vi "GOOP_Utility_IsClassVI.vi"(7 "KeepClassOpen(False)":bool, 8 "error in (no error)":errorcluster, 10 "ProjectItem":refnum<vi>, 11 "Object":u64) -> (0 "error out":errorcluster, 1 "ClassItem(If Found)":refnum<vi>, 2 "ClassProvider":string, 3 "Is Class VI?":bool, 4 "RootClassQualified Class Name":string, 5 "Is Interface?":bool)   [LabVIEW 2020]
uses:
  <resource>/Framework/Providers/Open_GDS/ClassProviders/Common/LvClass_class/GDSLvClass_ClassTypeSettingNames.ctl
  <resource>/Framework/Providers/Open_GDS/ClassProviders/Provider_LvNativeClass/LvNativeProviderName.ctl
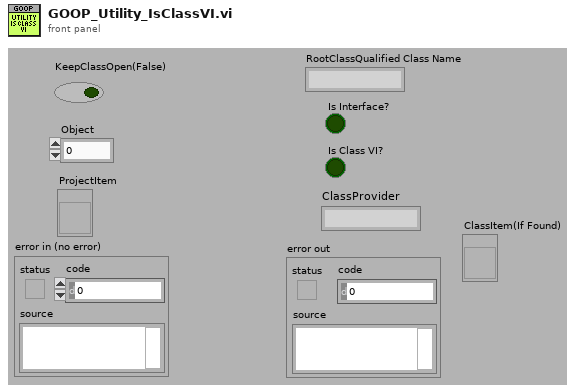
[diagram p1: front panel]
types:
  T1 = typedef "LvNativeProviderName.ctl" = enum16{"Endevo LabVIEW Native"}
  T2 = typedef "GDSLvClass_ClassTypeSettingNames.ctl" = enum16{"EndevoGOOP_ClassProvider", "EndevoGOOP_TemplateUsed", "EndevoGOOP_TemplateVersion", "EndevoGOOP_PlugIns", "EndevoGOOP_ConnectorPanePattern"}
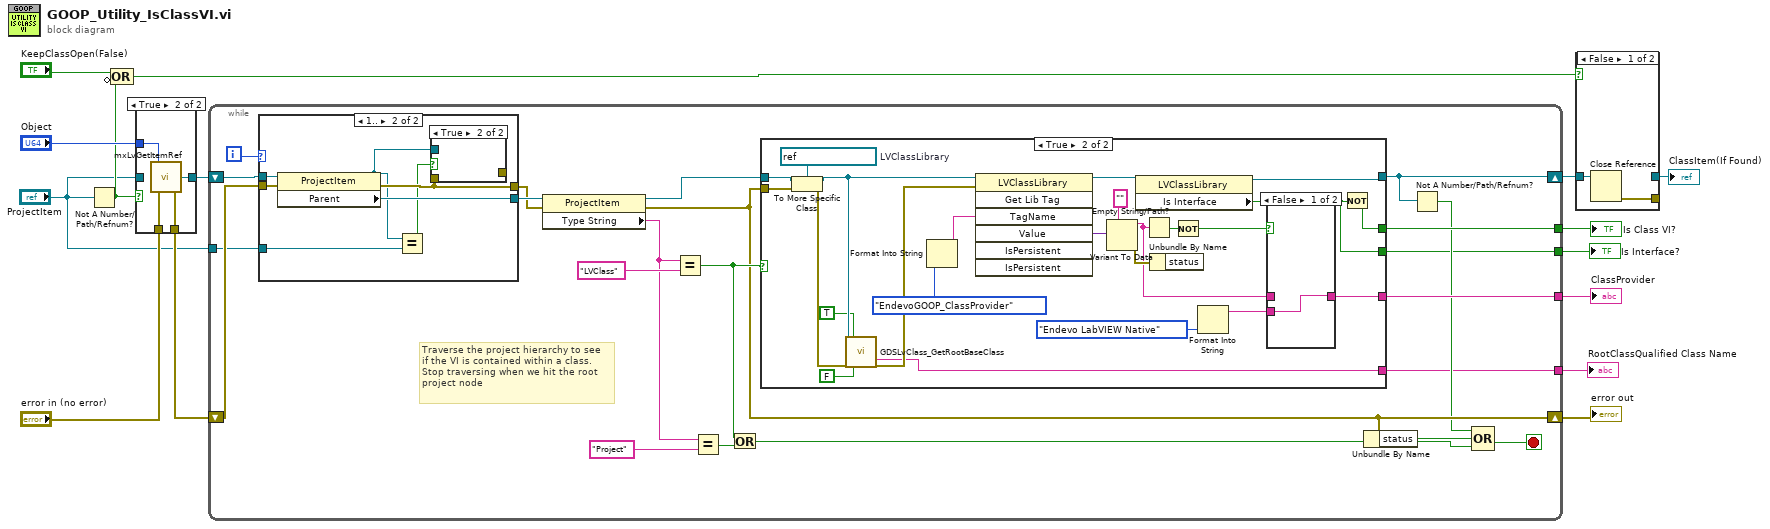
[diagram p0: block diagram]
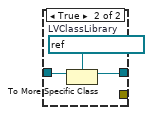
[diagram p3: hidden frame]
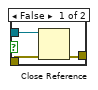
[diagram p5: hidden frame]
diagram:
  n1 = Not A Number/Path/Refnum?(number/path/refnum="ProjectItem") -> (NaN/Path/Refnum?=w4:bool)
  n2 = Compound Arithmetic op=OR("KeepClassOpen(False)", invert w4) -> (w5:bool)
  n3 = case shown="True" w4 {
    tunnel: "Object" -> [_ w21]
    tunnel: [w16 w20] -> w14
    tunnel: "error in (no error)" -> [w17 w19]
    tunnel: [w17 w18] -> w10
    tunnel: "ProjectItem" -> [w16 _]
    frame False {
    }
    frame True {
      n4 = call <resource>:"mxLvGetItemRef.vi"("Item"=w21, "error in"=w19) -> ("Item Refnum"=w20:refnum<vi>, "error out"=w18:errorcluster)  [unwired: 1 out]
    }
  }
  n5 = while {
    shift-right: [w29] -> w8
    shift-left: w14 -> [w41]
    tunnel: [w35] -> w13
    tunnel: [w34] -> w11
    shift-right: [w30] -> w9
    shift-left: w10 -> [w33]
    tunnel: "ProjectItem" -> [w24]
    tunnel: [w23] -> w2
    tunnel: [w22] -> w1
    i -> [w31]
    stop <- w25 stop-if-true
    # "Traverse the project hierarchy to see\nif the VI is contained within a class.\nStop traversing when we hit the root\nproject node"
    n6 = case shown="1.." w31 {
      tunnel: [w44 w52] -> w42
      tunnel: w41 -> [w44 w51]
      tunnel: w33 -> [w45 w50]
      tunnel: [w45 w49] -> w32
      tunnel: w24 -> [_ w47]
      frame Default {
      }
      frame 1.. {
        n7 = property class="ProjectItem"(reference=w51, error in=w50) -> (reference out=w48:refnum<vi>, error out=w49:errorcluster, "Parent"=w52:refnum<vi>)
        n8 = Equal?(x=w48, y=w47) -> (x = y?=w46:bool)
        n9 = case shown="True" w46 {
          tunnel: w49 -> [w55 _]
          tunnel: w48 -> [w54 _]
          tunnel: [w53 _] -> _
          frame False {
            n10 = Close Reference(reference=w54, error in (no error)=w55) -> (error out=w53:errorcluster)
          }
          frame True {
          }
        }
      }
    }
    n11 = property class="ProjectItem"(reference=w42, error in=w32) -> (reference out=w36:refnum<vi>, error out=w30:errorcluster, "Type String"=w39:string)
    n12 = Equal?(x=w39, y="LVClass") -> (x = y?=w37:bool)
    n13 = Equal?(x=w39, y="Project") -> (x = y?=w38:bool)
    n14 = Or(x=w37, y=w38) -> (x .or. y?=w26:bool)
    n15 = case shown="True" w37 {
      tunnel: w36 -> [w56 w80]
      tunnel: [w56 w59] -> w29
      tunnel: [_ w58] -> w35
      tunnel: [_ w68] -> w34
      tunnel: w30 -> [_ w75]
      tunnel: [_ w61] -> w23
      tunnel: [_ w57] -> w22
      frame False {
      }
      frame True {
        w79 = refnum<vi> refnum  # LVClassLibrary
        n16 = To More Specific Class(target class=w79, reference=w80, error in=w75) -> (specific class reference=w66:refnum<vi>, error out=w65:errorcluster)
        n17 = call <resource>:"GDSLvClass_GetRootBaseClass.vi"("ViRef/Path,LvClassRef/Path"=w66, "error in (no error)"=w65, "Don'tOpenReference"=TRUE, "LimitToSpecificProviderTypeOfSameType(True)"=FALSE) -> ("Qualified Class Name"=w61:string, "error out"=w64:errorcluster)  [unwired: 9 in, 5 out]
        n18 = Format Into String(GDSLvClass_ClassTypeSettingNames."EndevoGOOP_ClassProvider" ("ClassTypeSettingNames")) -> (resulting string=w74:string)  [unwired: 3 in, 1 out]
        n19 = invoke class="LVClassLibrary" method="Get Lib Tag"(reference=w66, error in=w64, "TagName"=w74) -> (reference out=w60:refnum<vi>, "Value"=w78:variant)  [unwired: 4 in, 5 out]
        n20 = Variant To Data(type="", Variant=w78) -> (data=w69:string, error out=w72:errorcluster)  [unwired: 1 in]
        n21 = property class="LVClassLibrary"(reference=w60) -> (reference out=w59:refnum<vi>, "Is Interface"=w57:bool)  [unwired: 1 in, 1 out]
        n22 = Empty String/Path?(string/path=w69) -> (empty?=w76:bool)
        n23 = Unbundle By Name(w72) -> ()  [unwired: 1 out]
        n24 = Not(x=w76) -> (.not. x?=w70:bool)
        n25 = Format Into String(LvNativeProviderName."Endevo LabVIEW Native" ("ProviderName")) -> (resulting string=w67:string)  [unwired: 3 in, 1 out]
        n26 = case shown="False" w70 {
          tunnel: w69 -> [_ w82]
          tunnel: [w81 w82] -> w68
          tunnel: w67 -> [w81 _]
          frame False {
          }
          frame True {
          }
        }
        n27 = Not(x=w57) -> (.not. x?=w58:bool)
      }
    }
    n28 = Unbundle By Name(w30) -> ("status"=w28:bool)
    n29 = Not A Number/Path/Refnum?(number/path/refnum=w29) -> (NaN/Path/Refnum?=w27:bool)
    n30 = Compound Arithmetic op=OR(w27, w28, w26) -> (w25:bool)
  }
  "Is Class VI?" <- w13
  "error out" <- w9
  "ClassProvider" <- w11
  "RootClassQualified Class Name" <- w2
  "Is Interface?" <- w1
  n31 = case shown="False" w5 {
    tunnel: w8 -> [w84 w86]
    tunnel: [_ w85] -> w6
    tunnel: [w83 _] -> _
    frame False {
      n32 = Close Reference(reference=w84) -> (error out=w83:errorcluster)  [unwired: 1 in]
    }
    frame True {
      w87 = refnum<vi> refnum  # LVClassLibrary
      n33 = To More Specific Class(target class=w87, reference=w86) -> (specific class reference=w85:refnum<vi>)  [unwired: 1 in, 1 out]
    }
  }
  "ClassItem(If Found)" <- w6
